vi "Property Tree Check Boxes.vi"() -> (1 "Checked":i32=38, 2 "Unchecked":i32=38, 3 "None":i32=37)   [LabVIEW 2023]
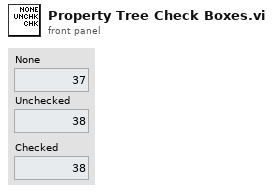
[diagram p1: front panel]
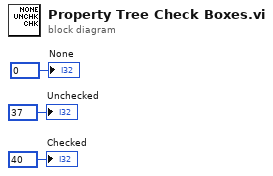
[diagram p0: block diagram]
diagram:
  "None" <- 0
  "Unchecked" <- 37
  "Checked" <- 40
